vi "S2DS_Save current user info (SubVI).vi"(4 "Logbook path":path, 5 "File index":u32, 6 "File prefix":string, 7 "Your email":string, 8 "error in (no error)":errorcluster, 9 "Current user":string, 10 "Session name":string, 11 "Project name":string) -> (0 "error out":errorcluster)   [LabVIEW 2025]
uses:
  <vilib>/Utility/config.llb/Write Key (String).vi
  <vilib>/Utility/config.llb/Write Key (U32).vi
  <vilib>/Utility/config.llb/Write Key (Path).vi
  <vilib>/Utility/config.llb/NI_LVConfig.lvlib
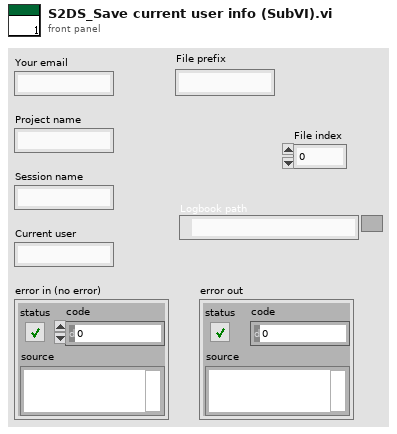
[diagram p1: front panel]
types:
  T1 = typedef "NI_LVConfig.lvlib/Config Data RefNum.ctl" = refnum<k1>
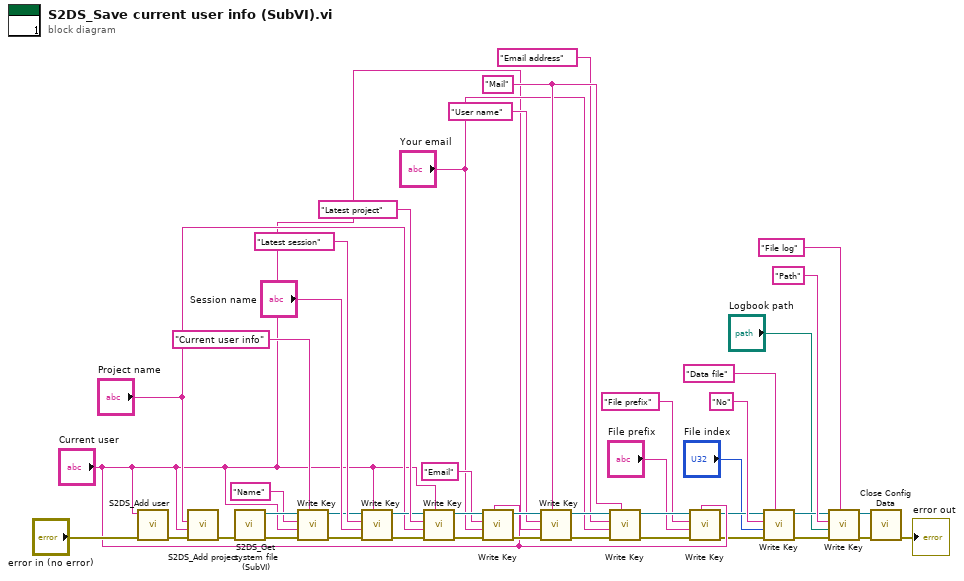
[diagram p0: block diagram]
diagram:
  w24 = "Mail" ("section")
  n1 = call "S2DS_Add user.vi"("error in (no error)"="error in (no error)", "new user"="Current user") -> ("error out"=w20:errorcluster)  [unwired: 9 in]
  n2 = call "S2DS_Add project.vi"("error in (no error)"=w20, "Your name"="Current user", "Add new project"="Project name") -> ("error out"=w19:errorcluster)  [unwired: 8 in]
  n3 = call "S2DS_Get system file (SubVI).vi"("error in (no error)"=w19) -> ("error out"=w34:errorcluster, "Refnum out"=w35:T1)  [unwired: 9 in]
  n4 = call-poly <vilib>:"Write Key.vi"("section"="Current user info", "error in (no error)"=w34, "value"="Current user", "key"="Name", "refnum"=w35) -> ("error out"=w30:errorcluster, "refnum out"=w31:T1)  [unwired: 4 in, 1 out]
  n5 = call-poly <vilib>:"Write Key.vi"("section"="Current user", "error in (no error)"=w30, "value"="Session name", "key"="Latest session", "refnum"=w31) -> ("error out"=w39:errorcluster, "refnum out"=w38:T1)  [unwired: 4 in, 1 out]
  n6 = call-poly <vilib>:"Write Key.vi"("section"="Current user", "error in (no error)"=w39, "value"="Project name", "key"="Latest project", "refnum"=w38) -> ("error out"=w43:errorcluster, "refnum out"=w42:T1)  [unwired: 4 in, 1 out]
  n7 = call-poly <vilib>:"Write Key.vi"("section"="Current user", "error in (no error)"=w43, "value"="Your email", "key"="Email", "refnum"=w42) -> ("error out"=w28:errorcluster, "refnum out"=w29:T1)  [unwired: 4 in, 1 out]
  n8 = call-poly <vilib>:"Write Key.vi"("section"=w24, "error in (no error)"=w28, "value"="Current user", "key"="User name", "refnum"=w29) -> ("error out"=w25:errorcluster, "refnum out"=w26:T1)  [unwired: 4 in, 1 out]
  n9 = call-poly <vilib>:"Write Key.vi"("section"=w24, "error in (no error)"=w25, "value"="Your email", "key"="Email address", "refnum"=w26) -> ("error out"=w16:errorcluster, "refnum out"=w17:T1)  [unwired: 4 in, 1 out]
  n10 = call-poly <vilib>:"Write Key.vi"("section"="Current user", "error in (no error)"=w16, "value"="File prefix", "key"="File prefix", "refnum"=w17) -> ("error out"=w10:errorcluster, "refnum out"=w9:T1)  [unwired: 4 in, 1 out]
  n11 = call-poly <vilib>:"Write Key.vi"("section"="Data file", "error in (no error)"=w10, "value"="File index", "key"="No", "refnum"=w9) -> ("error out"=w2:errorcluster, "refnum out"=w5:T1)  [unwired: 4 in, 1 out]
  n12 = call-poly <vilib>:"Write Key.vi"("section"="File log", "error in (no error)"=w2, "value"="Logbook path", "key"="Path", "refnum"=w5) -> ("error out"=w1:errorcluster, "refnum out"=w4:T1)  [unwired: 4 in, 1 out]
  n13 = call <vilib>:"Close Config Data.vi"("error in (no error)"=w1, "refnum"=w4) -> ("error out"=→"error out":errorcluster)  [unwired: 8 in, 1 out]
